vi "Image Tester[Circle].vi"(11 "Circle Descriptor":T1 {"Position"."Y" format="%.2f"; "Position"."X" format="%.2f"}) -> (3 "Positive":bool)   [LabVIEW 2016]
panel:
  in  "Particle Report":T2
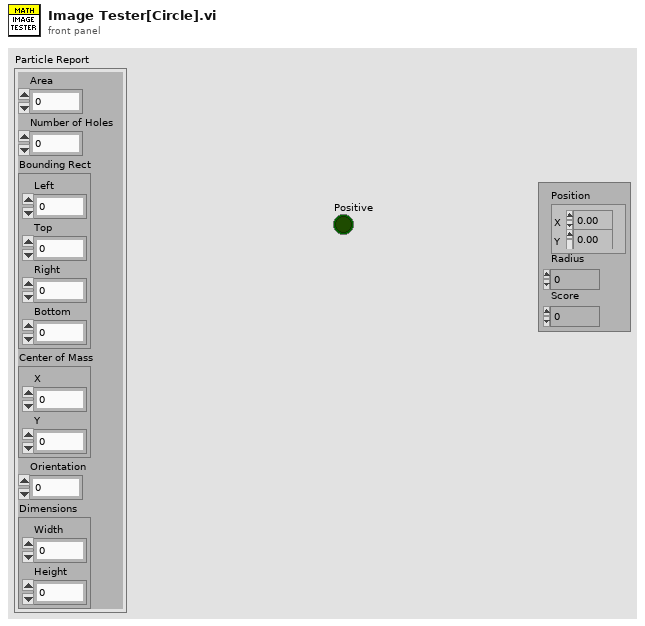
[diagram p1: front panel]
types:
  T1 = cluster{"Position":cluster{"X":sgl, "Y":sgl}, "Radius":dbl, "Score":dbl}
  T2 = cluster{"Area":dbl, "Number of Holes":dbl, "Bounding Rect":cluster{"Left":dbl, "Top":dbl, "Right":dbl, "Bottom":dbl}, "Center of Mass":cluster{"X":dbl, "Y":dbl}, "Orientation":dbl, "Dimensions":cluster{"Width":dbl, "Height":dbl}}
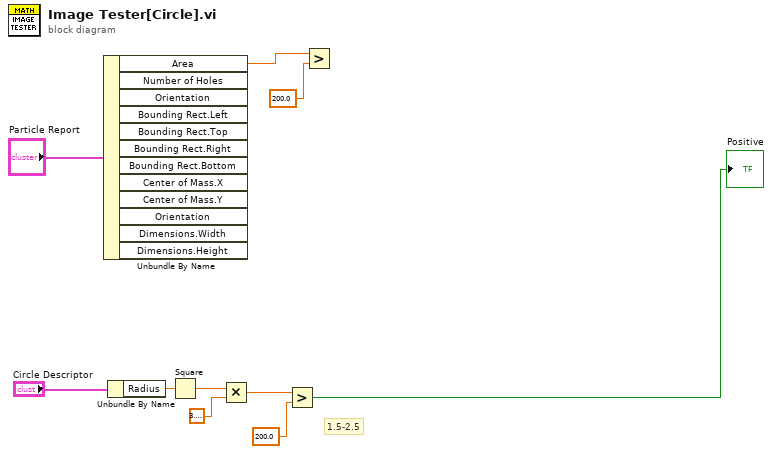
[diagram p0: block diagram]
diagram:
  # "1.5-2.5"
  n1 = Unbundle By Name("Particle Report") -> ("Area"=w8:dbl)  [unwired: 11 out]
  n2 = Unbundle By Name("Circle Descriptor") -> ("Radius"=w6:dbl)
  n3 = Square(x=w6) -> (x^2=w5:dbl)
  n4 = Multiply(x=w5, y=3.141592653589793) -> (x*y=w2:dbl)
  n5 = Greater?(x=w2, y=200.0 ("x")) -> (0:→"Positive":bool)
  n6 = Greater?(x=w8, y=200.0 ("x")) -> ()  [unwired: 1 out]
